vi "Add incoming ObjectInstance Record.vi"(8 "objectClassHandle":u64, 9 "objectInstanceHandle":u64, 10 "objectInstanceName":string, 11 "object instance records in":T1[](array[typedef])) -> (3 "object instance records out":T1[](array[typedef]))   [LabVIEW 2019, in "HLA Custom Device Engine.lvlib"]
uses:
  HLA Custom Device Engine.lvlib
  _typedefs/discoverObjectInstance_type.ctl
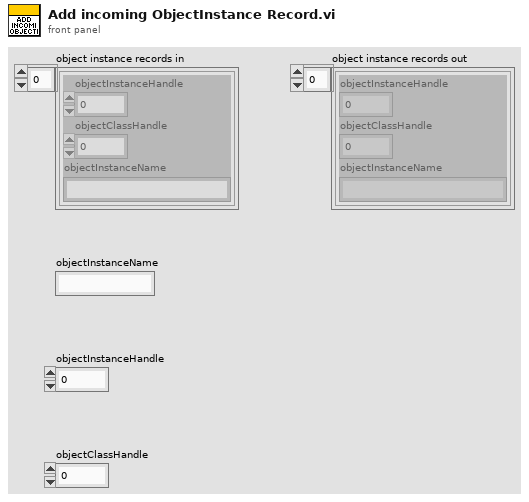
[diagram p1: front panel]
types:
  T1 = typedef "HLA Custom Device Engine.lvlib/discoverObjectInstance_type.ctl" = cluster{"objectInstanceHandle":u64, "objectClassHandle":u64, "objectInstanceName":string}
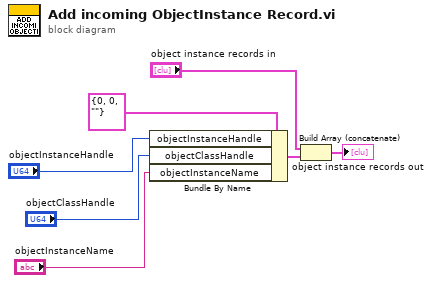
[diagram p0: block diagram]
diagram:
  n1 = Bundle By Name(cluster=T1 {"objectInstanceHandle"=0, "objectClassHandle"=0, "objectInstanceName"=""} ("discoverObjInstance_type"), "objectInstanceHandle"="objectInstanceHandle", "objectClassHandle"="objectClassHandle", "objectInstanceName"="objectInstanceName") -> (w7:T1)
  n2 = Build Array (concatenate)("object instance records in", w7) -> (→"object instance records out":T1[])
